vi "PT1000.vi"(1 "temperature \n(OR resistance)":dbl) -> (0 "resistance \n(OR temperature)":dbl)   [LabVIEW 2013]
panel:
  out "String":string="Pt1000"
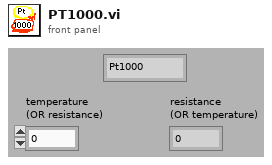
[diagram p1: front panel]
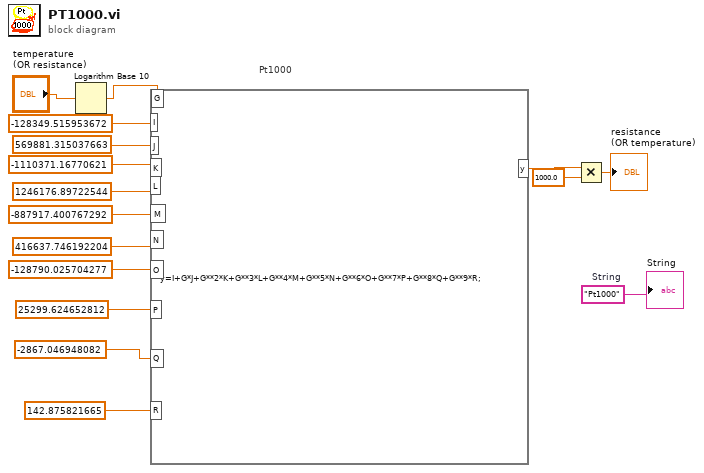
[diagram p0: block diagram]
diagram:
  w3 = "Pt1000"  # String
  # "Pt1000"
  n1 = Logarithm Base 10(1:"temperature \n(OR resistance)") -> (0:w15:dbl)
  n2 = formula code="y=I+G*J+G**2*K+G**3*L+G**4*M+G**5*N+G**6*O+G**7*P+G**8*Q+G**9*R;"("G"=w15, "I"=-128349.515953672 ("input variable"), "L"=1246176.89722544 ("input variable"), "M"=-887917.400767292 ("input variable"), "O"=-128790.025704277 ("input variable"), "Q"=-2867.046948082 ("input variable"), "R"=142.875821665 ("input variable"), "P"=25299.624652812 ("input variable"), "N"=416637.746192204 ("input variable"), "J"=569881.315037663 ("input variable"), "K"=-1110371.16770621 ("input variable")) -> ("y"=w14:dbl)
  n3 = Multiply(x=w14, y=1000.0) -> (x*y=→"resistance \n(OR temperature)":dbl)
  "String" <- w3
